vi "Read modbus.vi"(8 "error in (no error)":errorcluster, 11 "VISA Refnum in":refnum<visa-resource-name>) -> (0 "error out":errorcluster, 2 "read buffer":string, 3 "VISA Refnum out":refnum<visa-resource-name>)   [LabVIEW 2019]
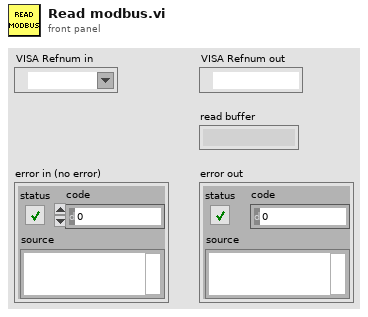
[diagram p1: front panel]
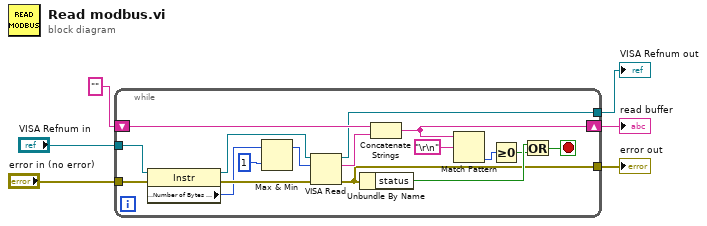
[diagram p0: block diagram]
diagram:
  n1 = while {
    tunnel: "VISA Refnum in" -> [w22]
    tunnel: "error in (no error)" -> [w20]
    shift-right: [w8] -> w6
    shift-left: "" ("write buffer") -> [w23]
    tunnel: [w9] -> w5
    tunnel: [w7] -> w4
    stop <- w18 stop-if-true
    n2 = property class="Instr"(reference=w22, error in=w20) -> (reference out=w21:refnum<visa-resource-name>, error out=w19:errorcluster, "Serial Settings:Number of Bytes at Serial Port"=w11:u32)
    n3 = Max & Min(x=w11, y=u32 1) -> (max(x,y)=w12:u32)  [unwired: 1 out]
    n4 = VISA Read(VISA resource name=w21, byte count=w12, error in (no error)=w19) -> (VISA resource name out=w7:refnum<visa-resource-name>, read buffer=w16:string, error out=w9:errorcluster)  [unwired: 1 out]
    n5 = Unbundle By Name(w9) -> ("status"=w17:bool)
    n6 = Concatenate Strings(w23, w16) -> (w8:string)
    n7 = Match Pattern(string=w8, regular expression="\r\n") -> (offset past match=w14:i32)  [unwired: 1 in, 3 out]
    n8 = Greater Or Equal To 0?(x=w14) -> (x >= 0?=w13:bool)
    n9 = Or(x=w17, y=w13) -> (x .or. y?=w18:bool)
  }
  "read buffer" <- w6
  "error out" <- w5
  "VISA Refnum out" <- w4
